vi "AngleStats_AngleResidual_BiFunc.vi"(9 "B":T1, 10 "A":T1, 11 "ExtraPassedData":variant) -> (0 "Error":bool, 3 "Result":T1)   [LabVIEW 2019, in "Trajectory_Library.lvlib"]
doc: "Returns a function that subtracts two vectors while normalizing the resulting value in the selected row as if it were an angle. The calling parameters for this function adhere to to those required to be called as F or H functions.\n \n\nInputs:\n - ExtraPassedData -- Extra data passed into this function. For this function, it contains: \n - angleStateIdx -- The row containing angles to be normalized.\n - A -- A matrix\n - B -- B matrix\n\nOutputs:\n - Result -- Function returning difference of two vectors with angle at the given index normalized.\n - Error -- If TRUE, an error occured."
uses:
  Trajectory_Library.lvlib
  <vilib>/Analysis/Matrix/Datatypes/RealMatrix.ctl
  <vilib>/Analysis/Matrix/NI_Matrix.lvlib
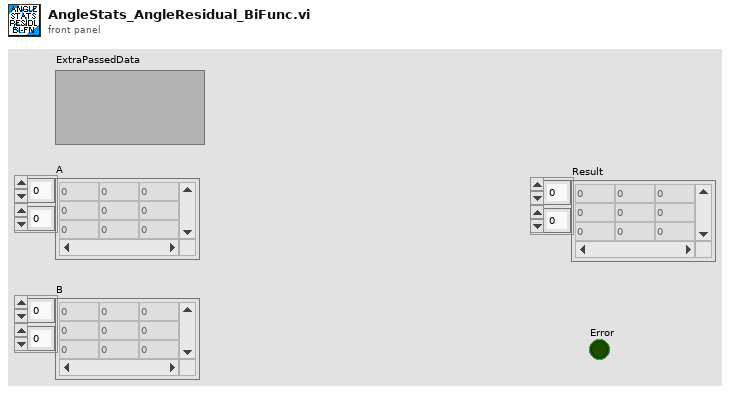
[diagram p1: front panel]
types:
  T1 = typedef "NI_Matrix.lvlib/RealMatrix.ctl" = dbl[][]
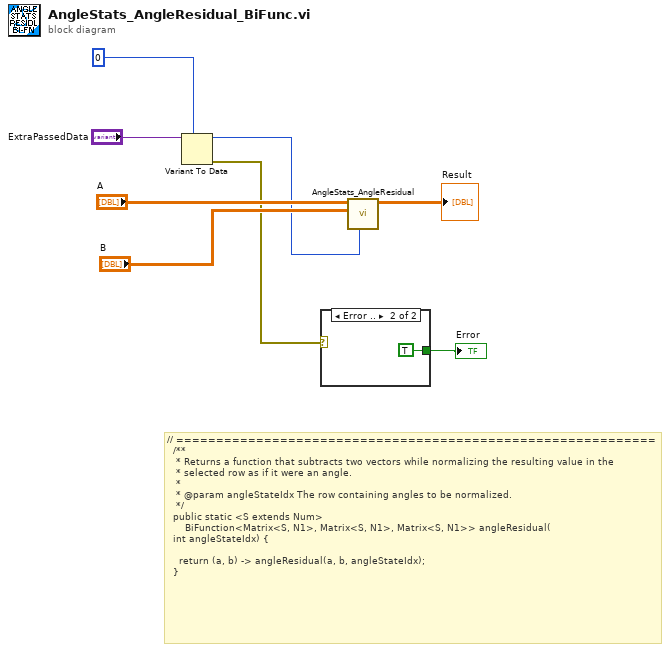
[diagram p0: block diagram]
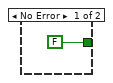
[diagram p2: hidden frame]
diagram:
  # "// ============================================================\n  /**\n   * Returns a function that subtracts two vectors while normalizing the resulting value in the\n   * selected row as if it were an angle.\n   *\n   * @param angleStateIdx The row containing angles to be normalized.\n   */\n  public static <S extends Num>\n      BiFunction<Matrix<S, N1>, Matrix<S, N1>, Matrix<S, N1>> angleResidual(\n\t\tint angleStateIdx) {\n\n    return (a, b) -> angleResidual(a, b, angleStateIdx);\n  }"
  n1 = Variant To Data(type=0, Variant="ExtraPassedData") -> (data=w4:i32, error out=w2:errorcluster)  [unwired: 1 in]
  n2 = case shown="Error .." w2 {
    tunnel: [FALSE TRUE] -> w1
    frame No Error {
    }
    frame Error {
    }
  }
  "Error" <- w1
  n3 = call "AngleStats_AngleResidual.vi"("Row"=w4, "B"="B", "A"="A") -> ("Result"=→"Result":T1)  [unwired: 8 in]
